vi "CONV String to 2D Boolean.vi"(0 "String":string, 1 "Delimiters (,;)":string=",;") -> (6 "2-D Boolean":bool[][](array[boolean]))   [LabVIEW 2012]
doc: "This routine converts a string list to a 2-D String Array. There should be exactly 2 characters in the Delimiters field. The first is the Column delimiter, and the Second is the Row delimiter.\n\nExample:\n\nString: 0,1,0;1,0,1\nDelimiters: ,;\n\nOutput\n\n0 1 0\n1 0 1"
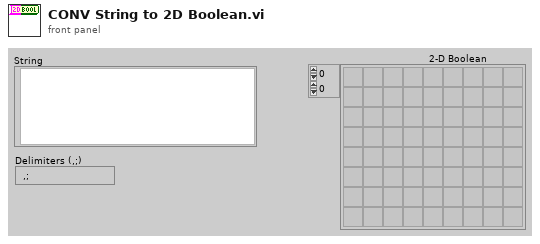
[diagram p1: front panel]
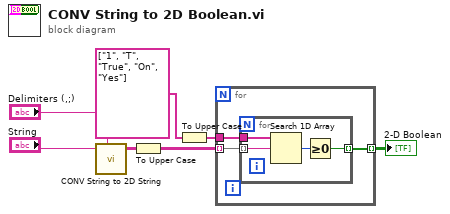
[diagram p0: block diagram]
diagram:
  n1 = call "CONV String to 2D String.vi"("String"="String", "Delimiters (,;)"="Delimiters (,;)") -> ("2-D String"=w5:string[][])  [unwired: 7 out]
  n2 = To Upper Case(1:w5) -> (0:w4:string[][])
  n3 = To Upper Case(1:string[] ["1", "T", "True", "On", "Yes"]) -> (0:w6:string[])
  n4 = for {
    tunnel: [w10] -> w1 mode=indexing
    tunnel: w6 -> [w9]
    tunnel: w4 -> [w8] mode=indexing
    n5 = for {
      tunnel: [w14] -> w10 mode=indexing
      tunnel: w9 -> [w12]
      tunnel: w8 -> [w11] mode=indexing
      n6 = Search 1D Array(1D array=w12, element=w11) -> (index of element=w13:i32)  [unwired: 1 in]
      n7 = Greater Or Equal To 0?(x=w13) -> (x >= 0?=w14:bool)
    }
  }
  "2-D Boolean" <- w1
